vi "SIM_Drive_ODOM_EXECUTE.vi"(8 "error in (no error)":errorcluster, 10 "module Positions":T1[](array[typedef]) {"Angle"."SIN" format="%13.4f"; "Angle"."COS" format="%13.4f"; "Angle"."VALUE" format="%13.4f"}, 11 "GyroAngleDeg":dbl) -> (0 "error out":errorcluster)   [LabVIEW 2023]
uses:
  <vilib>/Rock Robotics/WPI/ThirdParty/JAS_Junk/TrajLib/Rotation2d_Plus.vi
  <vilib>/Rock Robotics/WPI/ThirdParty/JAS_Junk/TrajLib/Twist2d_Create.vi
  <vilib>/Rock Robotics/WPI/ThirdParty/JAS_Junk/TrajLib/Rotation2d_Minus.vi
  <vilib>/Rock Robotics/WPI/ThirdParty/JAS_Junk/TrajLib/Pose2d_getTranslation.vi
  <vilib>/Rock Robotics/WPI/ThirdParty/JAS_Junk/TrajLib/Pose2d_New_TRRO.vi
  <vilib>/Rock Robotics/WPI/ThirdParty/JAS_Junk/TrajLib/VI/SwerveModulePosition_Get.vi
  <vilib>/Rock Robotics/WPI/ThirdParty/JAS_Junk/TrajLib/VI/SwerveModulePosition_New.vi
  <vilib>/Rock Robotics/WPI/ThirdParty/JAS_Junk/TrajLib/Twist2d_GetAll.vi
  <vilib>/Rock Robotics/WPI/ThirdParty/JAS_Junk/TrajLib/Rotation2d_RotateBy.vi
  <vilib>/Rock Robotics/WPI/ThirdParty/JAS_Junk/TrajLib/Rotation2d_UnaryMinus.vi
  <vilib>/Rock Robotics/WPI/ThirdParty/JAS_Junk/TrajLib/Rotation2d_CreateXY.vi
  <vilib>/Rock Robotics/WPI/ThirdParty/JAS_Junk/TrajLib/Util_CalcDist.vi
  SIM_Drive_Globals.vi
  <vilib>/Rock Robotics/WPI/ThirdParty/JAS_Junk/TrajLib/VI/SwerveKinematics_ToTwist2dX.vi
  <vilib>/Rock Robotics/WPI/ThirdParty/JAS_Junk/TrajLib/Pose2d_Exp.vi
  <vilib>/Rock Robotics/WPI/ThirdParty/JAS_Junk/TrajLib/Trajectory_Library.lvlib
  <vilib>/Rock Robotics/WPI/ThirdParty/JAS_Junk/TrajLib/TypeDef/ROTATION2D.ctl
  <vilib>/Rock Robotics/WPI/ThirdParty/JAS_Junk/TrajLib/TypeDef/SWERVE_DRIVE_MODULE_POSITION.ctl
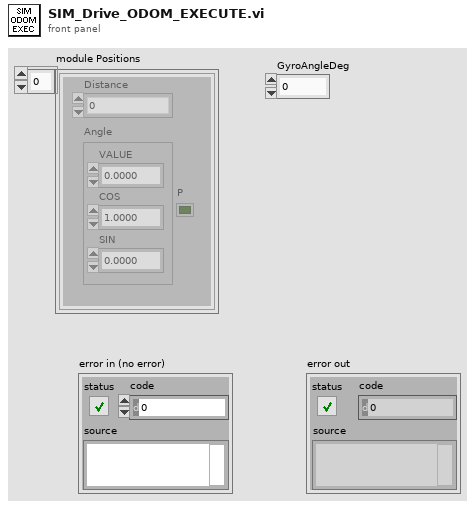
[diagram p1: front panel]
types:
  T1 = typedef "Trajectory_Library.lvlib/SWERVE_DRIVE_MODULE_POSITION.ctl" = cluster{"Distance":dbl, "Angle":T2, "P":bool}
  T2 = typedef "Trajectory_Library.lvlib/ROTATION2D.ctl" = cluster{"VALUE":dbl, "COS":dbl, "SIN":dbl}
  T3 = typedef "Trajectory_Library.lvlib/SWERVE_DRIVE_KINEMATICS.ctl" = cluster{"NumModules":i32, "InverseKinematics":T4, "ForwardKinematics":T4, "Modules":T5[], "PrevCoR":T5, "SavedModuleStates":T6[]}
  T4 = typedef "NI_Matrix.lvlib/RealMatrix.ctl" = dbl[][]
  T5 = typedef "Trajectory_Library.lvlib/TRANSLATION2D.ctl" = cluster{"X":dbl, "Y":dbl}
  T6 = typedef "Trajectory_Library.lvlib/SWERVE_DRIVE_MODULE_STATE.ctl" = cluster{"Speed":dbl, "Angle":T2}
  T7 = typedef "Trajectory_Library.lvlib/SWERVE_DRIVE_ODOMETRY.ctl" = cluster{"POSE":T8, "GyroOffset":T2, "PreviousAngle":T2, "PrevModulePositions":T1[], "NumModules":i32}
  T8 = typedef "Trajectory_Library.lvlib/POSE2D.ctl" = cluster{"TRANSLATION":T5, "ROTATION":T2}
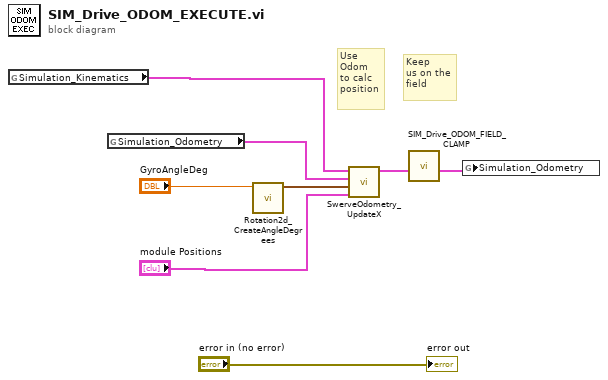
[diagram p0: block diagram]
diagram:
  # "Keep\nus on the\nfield"
  # "Use\nOdom\nto calc\nposition"
  n1 = global read "SIM_Drive_Globals.vi" "Simulation_Kinematics"() -> (w1:T3)
  n2 = global read "SIM_Drive_Globals.vi" "Simulation_Odometry"() -> (w5:T7)
  n3 = call <vilib>:"Rotation2d_CreateAngleDegrees.vi"("Angle_Degrees"="GyroAngleDeg") -> ("ROTATION"=w8:T2)  [unwired: 10 in]
  n4 = call <vilib>:"SwerveOdometry_UpdateX.vi"("module Positions"="module Positions", "gyroAngle"=w8, "in SWERVE_DRIVE_ODOMETRY"=w5, "SWERVE_DRIVE_KINEMATICS"=w1) -> ("out SWERVE_DRIVE_ODOMETRY"=w7:T7)  [unwired: 5 in, 2 out]
  n5 = call "SIM_Drive_ODOM_FIELD_CLAMP.vi"("in SWERVE_DRIVE_ODOMETRY"=w7) -> ("out SWERVE_DRIVE_ODOMETRY"=w4:T7)  [unwired: 10 in]
  n6 = global write "SIM_Drive_Globals.vi" "Simulation_Odometry"(w4) -> ()
  "error out" <- "error in (no error)"
